vi "appendix_writeReport.vi"(7 "AppendixTitle":string, 8 "error in (no error)":errorcluster, 9 "Precisions":i16[](array[numeric]), 10 "Data":T1[](array[typedef]), 11 "NI_report in":refnum<class "NI_report.lvclass">) -> (0 "error out":errorcluster, 3 "Report out":refnum<class "NI_report.lvclass">)   [LabVIEW 2016]
uses:
  <vilib>/Utility/NIReport.llb/NI_report.lvclass
  appendix_data.ctl
  WorReport_tableData.ctl
  WorReport_imageData.ctl
  <vilib>/Utility/NIReport.llb/HTML Report Image Alignment.ctl
  <vilib>/Utility/NIReport.llb/Append Image to Report (path wrap).vi
  <vilib>/addons/_office/word.llb/Word Easy Table (str).vi
  <vilib>/Utility/NIReport.llb/NI_ReportGenerationCore.lvlib
  <vilib>/addons/_office/NI_ReportGenerationToolkit.lvlib
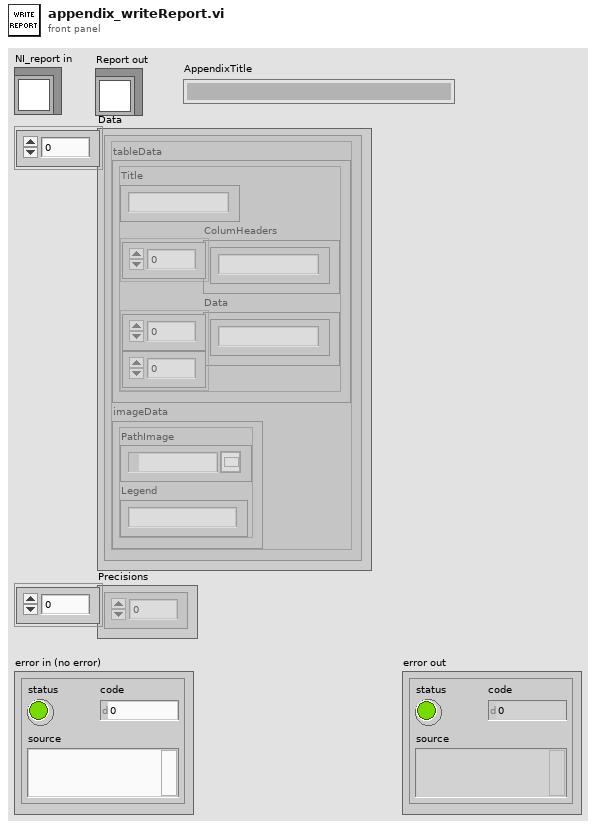
[diagram p1: front panel]
types:
  T1 = typedef "appendix_data.ctl" = cluster{"tableData":T2, "imageData":T3}
  T2 = typedef "WorReport_tableData.ctl" = cluster{"Title":string, "ColumHeaders":string[], "Data":string[][]}
  T3 = typedef "WorReport_imageData.ctl" = cluster{"PathImage":path, "Legend":string}
  T4 = typedef "NI_ReportGenerationCore.lvlib/HTML Report Image Alignment.ctl" = enum16{"(default)", "LEFT", "RIGHT", "TOP", "TEXTTOP", "MIDDLE", "ABSMIDDLE", "BASELINE", "BOTTOM", "ABSBOTTOM"}
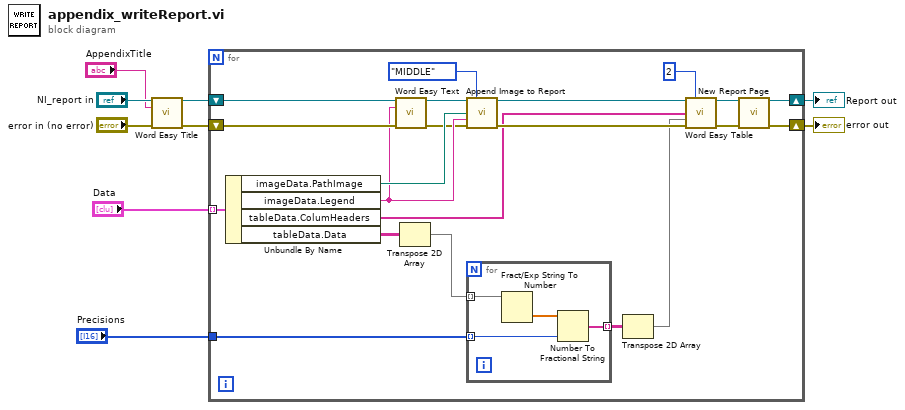
[diagram p0: block diagram]
diagram:
  n1 = call <vilib>:"Word Easy Title.vi"("report in"="NI_report in", "title"="AppendixTitle", "error in (no error)"="error in (no error)") -> ("report out"=w2:refnum<class "NI_report.lvclass">, "error out"=w4:errorcluster)  [unwired: 10 in, 1 out]
  n2 = for {
    tunnel: "Data" -> [w30] mode=indexing
    shift-right: [w15] -> w8
    shift-left: w4 -> [w28]
    shift-right: [w16] -> w6
    shift-left: w2 -> [w27]
    tunnel: "Precisions" -> [w11]
    n3 = Unbundle By Name(w30) -> ("imageData.PathImage"=w29:path, "imageData.Legend"=w25:string, "tableData.ColumHeaders"=w20:string[], "tableData.Data"=w14:string[][])
    n4 = call <vilib>:"Word Easy Text.vi"("report in"=w27, "text"=w25, "error in (no error)"=w28) -> ("report out"=w24:refnum<class "NI_report.lvclass">, "error out"=w23:errorcluster)  [unwired: 10 in, 1 out]
    n5 = Transpose 2D Array(2D array=w14) -> (transposed array=w13:string[][])
    n6 = call-poly <vilib>:"Append Image to Report.vi"("report in"=w24, "alignment (default)"=HTML_Report_Image_Alignment."MIDDLE", "path or URL of image"=w29, "caption or alternative string"=w25, "error in (no error)"=w23) -> ("report out"=w21:refnum<class "NI_report.lvclass">, "error out"=w22:errorcluster)  [unwired: 7 in, 2 out]
    n7 = for {
      tunnel: w13 -> [w34] mode=indexing
      tunnel: w11 -> [w32] mode=indexing
      tunnel: [w31] -> w12 mode=indexing
      n8 = Fract/Exp String To Number(string=w34) -> (number=w33:dbl[])  [unwired: 3 in, 1 out]
      n9 = Number To Fractional String(number=w33, precision (6)=w32) -> (F-format string=w31:string[])  [unwired: 2 in]
    }
    n10 = Transpose 2D Array(2D array=w12) -> (transposed array=w10:string[][])
    n11 = call-poly <vilib>:"Word Easy Table.vi"("report in"=w21, "auto format (none)"=2, "column headers"=w20, "data"=w10, "error in (no error)"=w22) -> ("report out"=w17:refnum<class "NI_report.lvclass">, "error out"=w18:errorcluster)  [unwired: 8 in, 1 out]
    n12 = call-dynamic "New Report Page.vi"("report in"=w17, "error in (no error)"=w18) -> ("report out"=w16:refnum<class "NI_report.lvclass">, "error out"=w15:errorcluster)  [unwired: 12 in]
  }
  "error out" <- w8
  "Report out" <- w6
